vi "Write I8.vi"(8 "error in":errorcluster, 9 "value in":i8, 10 "register name":string, 11 "session in":u32) -> (0 "error out":errorcluster, 3 "session out":u32)   [LabVIEW 2020, in "FPGA Register IO.lvlib"]
uses:
  FPGA Register IO.lvlib
  SubVIs/Check Register Data Store.vi
  Error Handling/Error 6001.vi
  Error Handling/Error 6000.vi
  Error Handling/Error 6002.vi
  NiFpga.dll
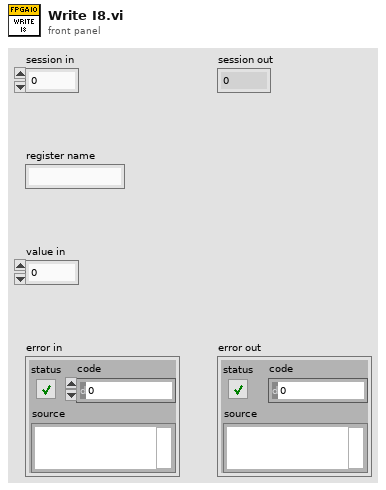
[diagram p1: front panel]
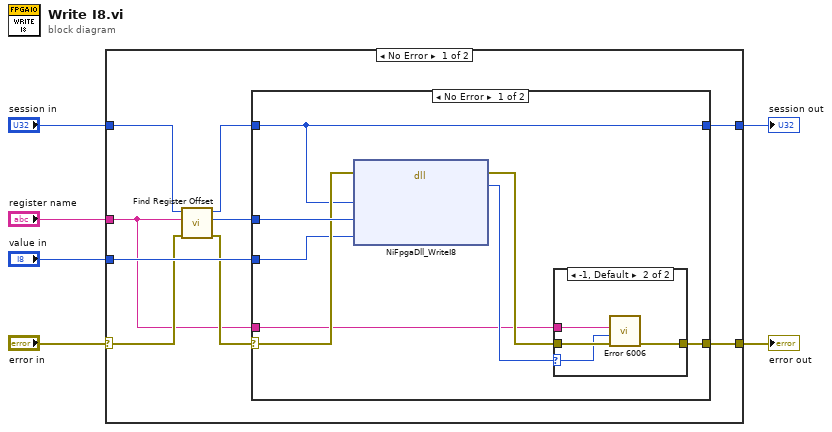
[diagram p0: block diagram]
diagram:
  n1 = case shown="No Error" "error in" {
    selector: "error in" -> [w11 w31]
    tunnel: "session in" -> [w12 w32]
    tunnel: [w15 w31] -> w5
    tunnel: [w14 w32] -> w4
    tunnel: "value in" -> [w13 _]
    tunnel: "register name" -> [w7 _]
    frame No Error {
      n2 = call "Find Register Offset.vi"("error in (no error)"=w11, "register name"=w7, "session in"=w12) -> ("error out"=w10:errorcluster, "resource offset"=w9:u32, "session out"=w8:u32)  [unwired: 6 in]
      n3 = case shown="No Error" w10 {
        selector: w10 -> [w22 w30]
        tunnel: w8 -> [w21 w29]
        tunnel: [w16 w30] -> w15
        tunnel: w9 -> [w23 _]
        tunnel: [w21 w29] -> w14
        tunnel: w13 -> [w20 _]
        tunnel: w7 -> [w17 _]
        frame No Error {
          n4 = dll-call lib="NiFpga.*" fn="NiFpgaDll_WriteI8"(error in=w22, "session"=w21, "offset"=w23, "value"=w20) -> (error out=w18:errorcluster, "status"=w19:i32)  [unwired: 5 in, 1 out]
          n5 = case shown="-1, Default" w19 {
            selector: w19 -> [_ w25]
            tunnel: w18 -> [w24 w26]
            tunnel: [w24 w28] -> w16
            tunnel: w17 -> [_ w27]
            frame 0 {
            }
            frame -1, Default {
              n6 = call "Error 6006.vi"("error in (no error)"=w26, "rio status code"=w25, "register name"=w27) -> ("error out"=w28:errorcluster)  [unwired: 8 in]
            }
          }
        }
        frame Error {
        }
      }
    }
    frame Error {
    }
  }
  "error out" <- w5
  "session out" <- w4
